vi "NI VeriStand - Set Custom Device Waveform Units.vi"(8 "error in (no error)":errorcluster, 10 "Units":string, 11 "Waveform Ref in":T1 format="%.0x") -> (0 "error out":errorcluster, 3 "Waveform Ref out":T1=18446744073709551615 format="%.0x")   [LabVIEW 2020, in "Custom Device API.lvlib"]
doc: "Sets the units of measurement for a waveform. Units can be any string that makes sense for your custom device."
uses:
  <vilib>/NI VeriStand/Custom Device API/Custom Device API.lvlib
  <vilib>/NI VeriStand/Custom Device API/Custom Device Item Ref.ctl
  7d8f2cef-580b-4e84-afef-6edd63e3a8fa.vi
  <vilib>/NI VeriStand/Custom Device API/Custom Device Offline Path.vi
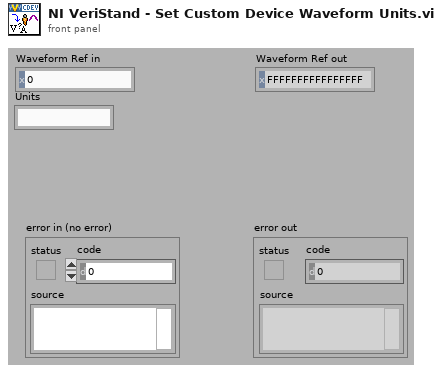
[diagram p1: front panel]
types:
  T1 = typedef "Custom Device API.lvlib/Custom Device Item Ref.ctl" = u64
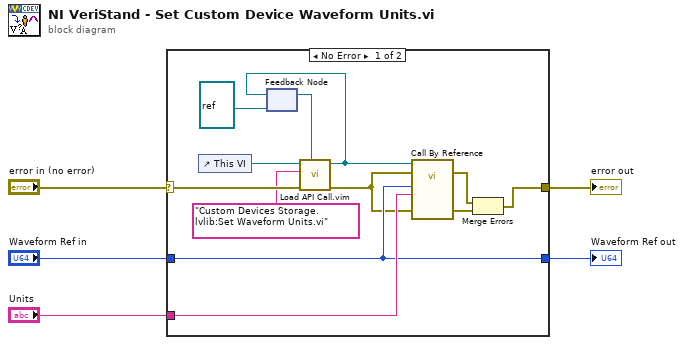
[diagram p0: block diagram]
diagram:
  n1 = case shown="No Error" "error in (no error)" {
    selector: "error in (no error)" -> [w11 w19]
    tunnel: [w16 w19] -> w5
    tunnel: "Waveform Ref in" -> [w14 w18]
    tunnel: [w14 w18] -> w3
    tunnel: "Units" -> [w15 _]
    frame No Error {
      n2 = control-ref of="This VI"() -> (w12:refnum<vi>)
      n3 = feedback #1(refnum<vi> refnum ("type specifier VI Refnum (for type only)")) -> (w13:refnum<vi>)
      n4 = call "Load API Call.vim"("VI reference in"=w13, "error in (no error)"=w11, "VI qualified name"="Custom Devices Storage.lvlib:Set Waveform Units.vi", "Caller VI ref"=w12) -> ("error out"=w7:errorcluster, "VI reference"=w10:refnum<vi>)  [unwired: 6 in]
      n5 = feedback-in #1(w10) -> ()
      n6 = call-by-ref "?"(reference=w10, error in=w7, 8:"error in (no error)"=w7, "Units"=w15, "Waveform Ref in"=w14) -> (error out=w6:errorcluster, 0:"error out"=w17:errorcluster)  [unwired: 7 in, 2 out]
      n7 = Merge Errors(w6, w17) -> (w16:errorcluster)
    }
    frame Error {
    }
  }
  "error out" <- w5
  "Waveform Ref out" <- w3
